vi "Configure Acquisition Sample Rate.vi"(6 "Setting Type (0: Analog)":u16(ring) items=["Analog", "Digital"], 7 "Sample Rate (0)":dbl, 8 "error in (no error)":errorcluster, 9 "Automatic Sampling Rate (T: Enable)":bool=TRUE, 10 "Sample Rate Method (0: Auto)":i32(ring) items=["Auto", "Max", "Manual"], 11 "VISA resource name":refnum<visa-resource-name>) -> (0 "error out":errorcluster, 3 "VISA resource name out":refnum<visa-resource-name>)   [LabVIEW 2020, in "Agilent 90000 Series.lvlib"]
doc: "Configures the settings of acquisition sample rate."
uses:
  Agilent 90000 Series.lvlib
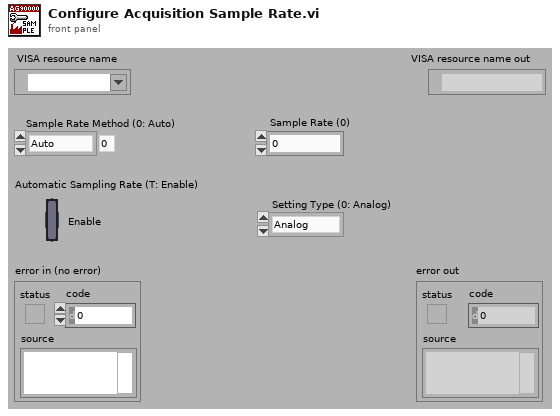
[diagram p1: front panel]
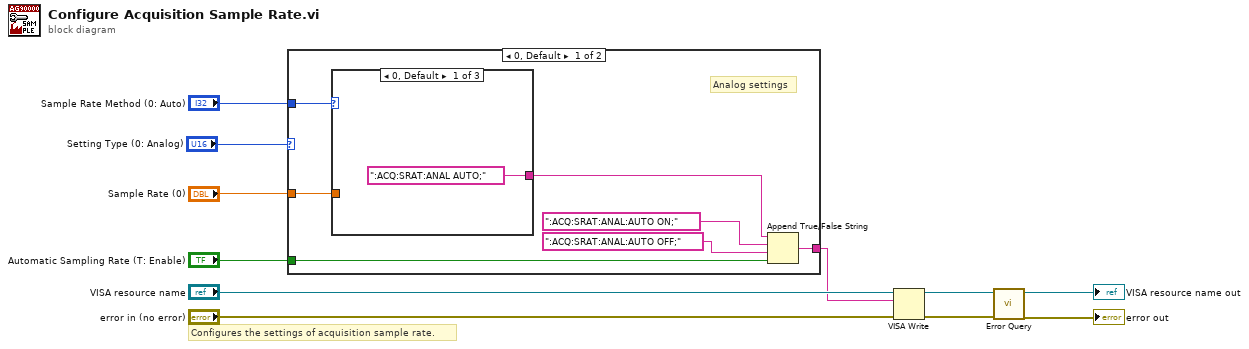
[diagram p0: block diagram]
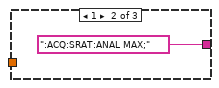
[diagram p2: hidden frame]
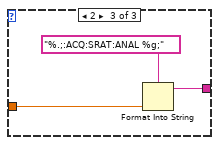
[diagram p3: hidden frame]
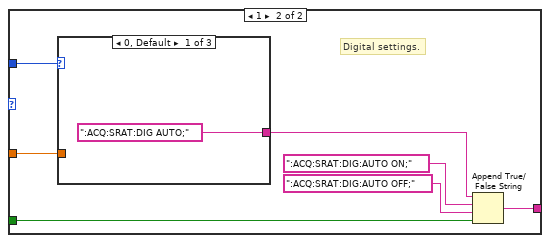
[diagram p4: hidden frame]
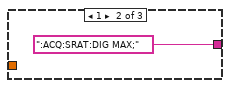
[diagram p5: hidden frame]
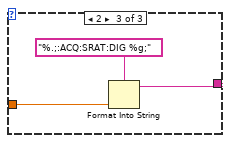
[diagram p6: hidden frame]
diagram:
  # "Configures the settings of acquisition sample rate."
  n1 = case shown="0, Default" "Setting Type (0: Analog)" {
    tunnel: "Sample Rate Method (0: Auto)" -> [w18 w30]
    tunnel: "Automatic Sampling Rate (T: Enable)" -> [w13 w26]
    tunnel: "Sample Rate (0)" -> [w15 w29]
    tunnel: [w12 w24] -> w1
    frame 0, Default {
      # "Analog settings"
      n2 = case shown="0, Default" w18 {
        tunnel: w15 -> [_ _ w22]
        tunnel: [":ACQ:SRAT:ANAL AUTO;" ":ACQ:SRAT:ANAL MAX;" w21] -> w14
        frame 0, Default {
        }
        frame 1 {
        }
        frame 2 {
          n3 = Format Into String(format string="%.;:ACQ:SRAT:ANAL %g;", w22) -> (resulting string=w21:string)  [unwired: 2 in, 1 out]
        }
      }
      n4 = Append True/False String(1:w13, 2:":ACQ:SRAT:ANAL:AUTO OFF;", 3:":ACQ:SRAT:ANAL:AUTO ON;", 4:w14) -> (0:w12:string)
    }
    frame 1 {
      # "Digital settings."
      n5 = case shown="0, Default" w30 {
        tunnel: w29 -> [_ _ w34]
        tunnel: [":ACQ:SRAT:DIG AUTO;" ":ACQ:SRAT:DIG MAX;" w33] -> w25
        frame 0, Default {
        }
        frame 1 {
        }
        frame 2 {
          n6 = Format Into String(format string="%.;:ACQ:SRAT:DIG %g;", w34) -> (resulting string=w33:string)  [unwired: 2 in, 1 out]
        }
      }
      n7 = Append True/False String(1:w26, 2:":ACQ:SRAT:DIG:AUTO OFF;", 3:":ACQ:SRAT:DIG:AUTO ON;", 4:w25) -> (0:w24:string)
    }
  }
  n8 = VISA Write(VISA resource name="VISA resource name", write buffer=w1, error in (no error)="error in (no error)") -> (VISA resource name out=w9:refnum<visa-resource-name>, error out=w8:errorcluster)  [unwired: 1 out]
  n9 = call "Error Query.vi"("error in (no error)"=w8, "VISA resource name"=w9) -> ("error out"=→"error out":errorcluster, "VISA resource name out"=→"VISA resource name out":refnum<visa-resource-name>)  [unwired: 8 out]
